vi "Get Named Nested Tag.vi"(8 "error in (no error)":errorcluster, 10 "Path":cluster{"Tag Name":string, "Index":i32}[](array[cluster]), 11 "Raw Message in":refnum<class "Raw Message.lvclass">) -> (0 "error out":errorcluster, 2 "Nested Message":refnum<class "Raw Message.lvclass">, 3 "Raw Message out":refnum<class "Raw Message.lvclass">)   [LabVIEW 2020]
uses:
  Raw Message.lvclass/Raw Message.ctl
  Raw Message.lvclass
  E:/Labview/LV 2020/Libs/LV Protobuf Raw/Source/Tag/Basic Type.lvclass
  E:/Labview/LV 2020/Libs/LV Protobuf Raw/Source/Proto Value/Proto Type.lvclass
  E:/Labview/LV 2020/Libs/LV Protobuf Raw/Source/Type Serializer/Type Serializer.lvclass
  E:/Labview/LV 2020/Libs/LV Protobuf Raw/Source/String Representable/String Representable.lvclass
  E:/Labview/LV 2020/Libs/LV Protobuf Raw/Source/Wire Type Group/Wire Type Group.lvclass
  E:/Labview/LV 2020/Libs/LV Protobuf Raw/Source/LEN Encoder/LEN.lvclass
  E:/Labview/LV 2020/Libs/LV Protobuf Raw/Source/Message/Raw Message.lvclass
  Tag/Basic Type.lvclass
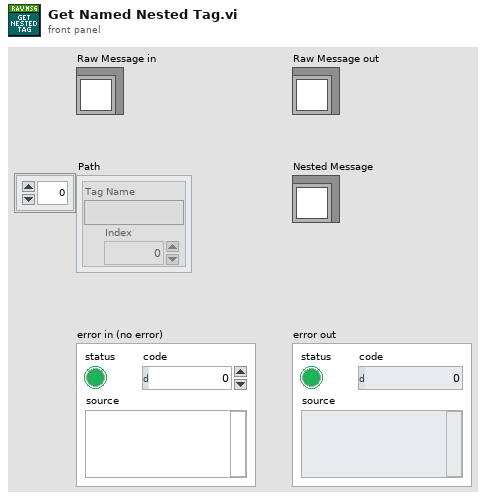
[diagram p1: front panel]
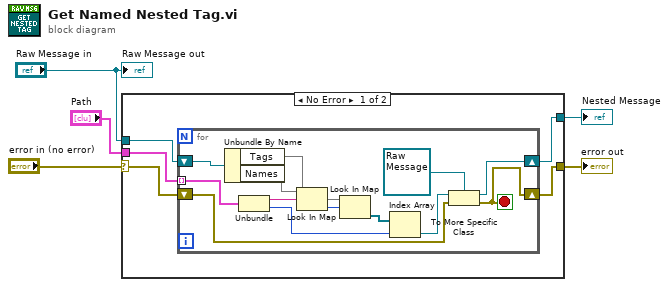
[diagram p0: block diagram]
diagram:
  n1 = case shown="No Error" "error in (no error)" {
    selector: "error in (no error)" -> [w7 w24]
    tunnel: [w10 w24] -> w5
    tunnel: [w9 _] -> w4
    tunnel: "Path" -> [w8 _]
    tunnel: "Raw Message in" -> [w6 _]
    frame No Error {
      n2 = for {
        shift-right: [w14] -> w10
        shift-left: w7 -> [w23]
        tunnel: w8 -> [w22] mode=indexing
        shift-right: [w15] -> w9
        shift-left: w6 -> [w21]
        stop <- w14 stop-if-true
        n3 = Unbundle By Name(w21) -> ("Tags"=w20, "Names"=w13)
        n4 = Unbundle(w22) -> ("Tag Name"=w12:string, "Index"=w18:i32)
        n5 = Look In Map(map=w13, key=w12) -> (value=w11:u32)  [unwired: 1 in, 1 out]
        n6 = Look In Map(map=w20, key=w11) -> (value=w19:refnum<class "Basic Type.lvclass">[])  [unwired: 1 in, 1 out]
        n7 = Index Array(array=w19, index=w18) -> (element=w17:refnum<class "Basic Type.lvclass">)
        n8 = To More Specific Class(target class=refnum<class "Raw Message.lvclass"> refnum ("Raw Message in"), reference=w17, error in=w23) -> (specific class reference=w15:refnum<class "Raw Message.lvclass">, error out=w14:errorcluster)
      }
    }
    frame Error {
    }
  }
  "error out" <- w5
  "Nested Message" <- w4
  "Raw Message out" <- "Raw Message in"
